vi "elog_text.vi"(7 "reply?":bool, 8 "error in (no error)":errorcluster, 9 "Num ID to reply":string, 10 "Text to log":string="reply a terzo testo da labview per elog", 11 "Elog Properties":T5={"Logbook"="CTS", "Author"="Hampai", "Type"="Experiment", "Category"="General", "Severity"="Log"}) -> (0 "error out":errorcluster)   [LabVIEW 2022 SP3]
uses:
  global/elog global.vi
  control/logbook.ctl
  control/type.ctl
  control/category.ctl
  control/severity.ctl
panel:
  out "resulting string":string
  out "return code":i32
  out "standard error":string
  out "standard output":string
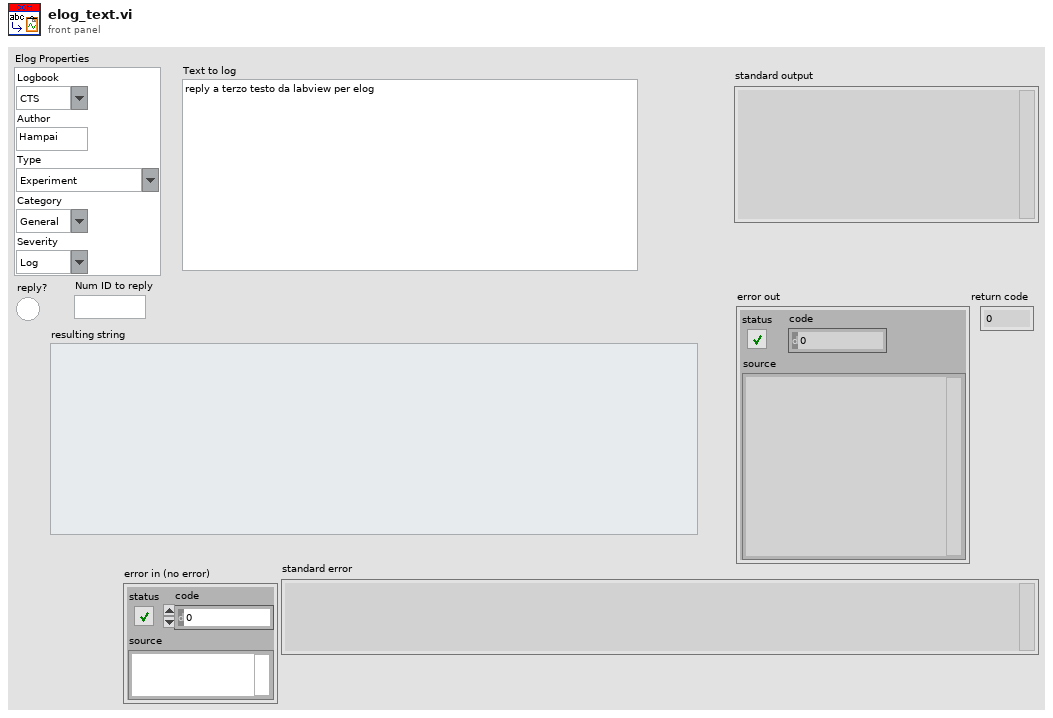
[diagram p1: front panel]
types:
  T1 = typedef "logbook.ctl" = string
  T2 = typedef "type.ctl" = string
  T3 = typedef "category.ctl" = string
  T4 = typedef "severity.ctl" = string
  T5 = cluster{"Logbook":T1, "Author":string, "Type":T2, "Category":T3, "Severity":T4}
  T6 = enum16{"open", "replace", "create", "open or create", "replace or create", "replace or create with confirmation"}
  T7 = cluster{"Complete Path Elog Exec":string, "IP Address Server Elog":string, "Port Server Elog":string}
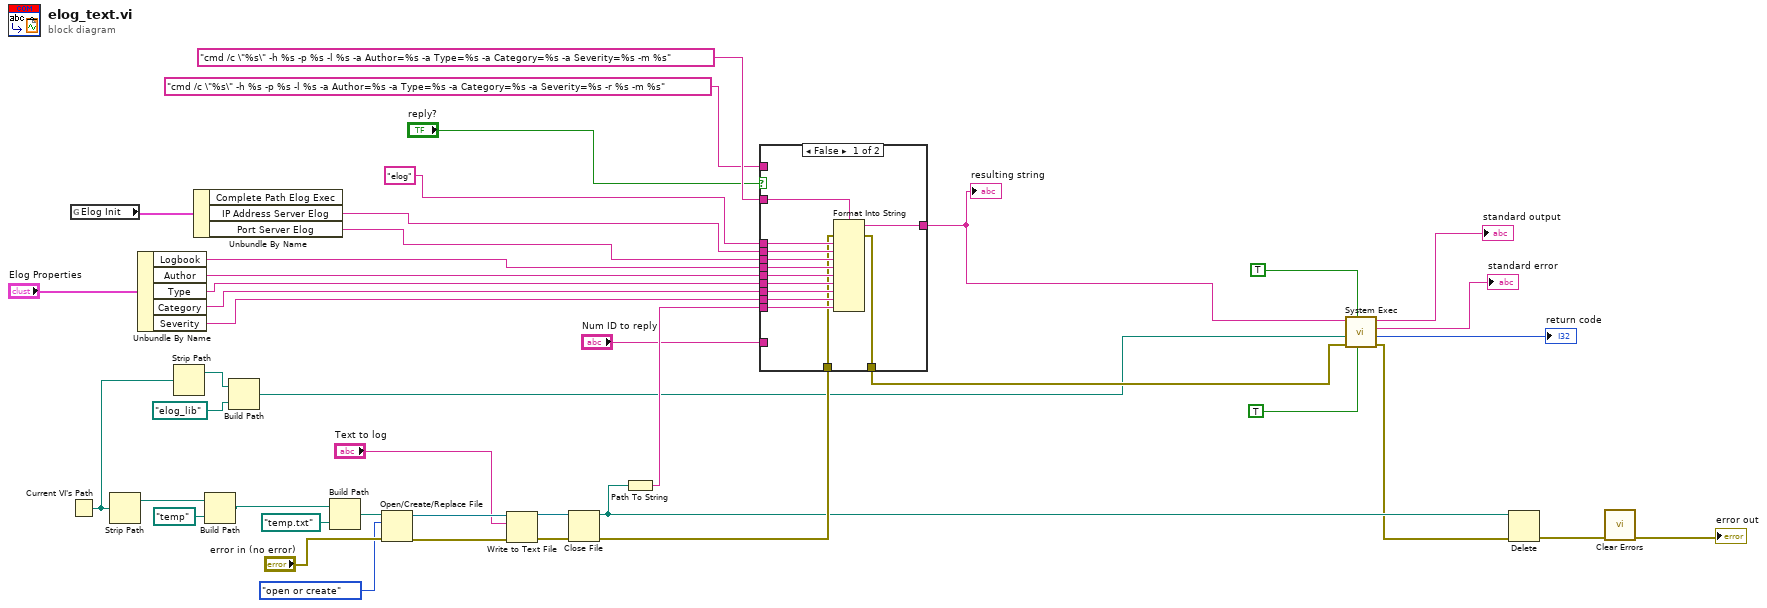
[diagram p0: block diagram]
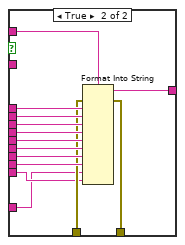
[diagram p2: hidden frame]
diagram:
  n1 = Current VI's Path() -> (path=w4:path)
  n2 = global read "elog global.vi" "Elog Init"() -> (w11:T7)
  n3 = Strip Path(path=w4) -> (stripped path=w8:path)  [unwired: 1 out]
  n4 = Unbundle By Name("Elog Properties") -> ("Logbook"=w18:T1, "Author"=w17:string, "Type"=w16:T2, "Category"=w15:T3, "Severity"=w14:T4)
  n5 = Strip Path(path=w4) -> (stripped path=w3:path)  [unwired: 1 out]
  n6 = Unbundle By Name(w11) -> ("IP Address Server Elog"=w10:string, "Port Server Elog"=w9:string)  [unwired: 1 out]
  n7 = Build Path(base path=w8, name or relative path=path "temp") -> (appended path=w6:path)
  n8 = Build Path(base path=w3, name or relative path=path "elog_lib") -> (appended path=w1:path)
  n9 = Build Path(base path=w6, name or relative path=path "temp.txt") -> (appended path=w28:path)
  n10 = Open/Create/Replace File(file path (use dialog)=w28, error in="error in (no error)", operation (0:open)=T6."open or create") -> (refnum out=w34:refnum<file>, error out=w32:errorcluster)  [unwired: 3 in, 1 out]
  n11 = Write to Text File(file (use dialog)=w34, text="Text to log", error in=w32) -> (refnum out=w30:refnum<file>, error out=w29:errorcluster)  [unwired: 1 in, 1 out]
  n12 = Close File(refnum=w30, error in=w29) -> (path=w25:path, error out=w26:errorcluster)
  n13 = Path To String(path=w25) -> (string=w31:string)
  n14 = case shown="False" "reply?" {
    tunnel: "cmd /c \"%s\" -h %s -p %s -l %s -a Author=%s -a Type=%s -a Category=%s -a Severity=%s -m %s" ("format string") -> [w56 _]
    tunnel: "elog" -> [w55 w70]
    tunnel: w10 -> [w54 w69]
    tunnel: w9 -> [w53 w68]
    tunnel: w18 -> [w52 w67]
    tunnel: w17 -> [w51 w66]
    tunnel: w16 -> [w50 w65]
    tunnel: w15 -> [w49 w64]
    tunnel: w14 -> [w48 w63]
    tunnel: [w47 w62] -> w37
    tunnel: w31 -> [w46 w58]
    tunnel: w26 -> [w45 w61]
    tunnel: [w44 w60] -> w23
    tunnel: "cmd /c \"%s\" -h %s -p %s -l %s -a Author=%s -a Type=%s -a Category=%s -a Severity=%s -r %s -m %s" ("format string") -> [_ w59]
    tunnel: "Num ID to reply" -> [_ w57]
    frame False {
      n15 = Format Into String(format string=w56, error in=w45, w55, w54, w53, w52, w51, w50, w49, w48, w46) -> (resulting string=w47:string, error out=w44:errorcluster)  [unwired: 1 in]
    }
    frame True {
      n16 = Format Into String(format string=w59, error in=w61, w70, w69, w68, w67, w66, w65, w64, w63, w57, w58) -> (resulting string=w62:string, error out=w60:errorcluster)  [unwired: 1 in]
    }
  }
  "resulting string" <- w37
  n17 = call <vilib>:"System Exec.vi"("run minimized? (F)"=TRUE, "wait until completion? (T)"=TRUE, "error in (no error)"=w23, "working directory"=w1, "command line"=w37) -> ("error out"=w24:errorcluster, "return code"=→"return code":i32, "standard error"=→"standard error":string, "standard output"=→"standard output":string)  [unwired: 3 in]
  n18 = Delete(path (use dialog)=w25, error in=w24) -> (error out=w13:errorcluster)  [unwired: 3 in, 2 out]
  n19 = call <vilib>:"Clear Errors.vi"("error in (no error)"=w13) -> ("error out"=→"error out":errorcluster)  [unwired: 5 in, 1 out]
